vi "Peregrine_close.vi"(2 "error in (no error)":errorcluster, 3 "Handle in":refnum<visa-resource-name>) -> (0 "error out":errorcluster)   [LabVIEW 2019]
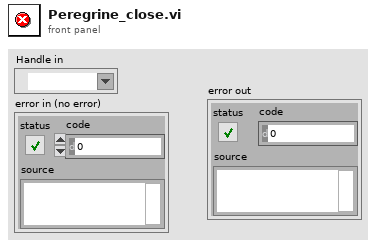
[diagram p1: front panel]
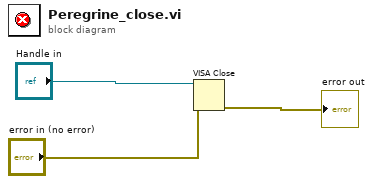
[diagram p0: block diagram]
diagram:
  n1 = VISA Close(VISA resource name="Handle in", error in (no error)="error in (no error)") -> (error out=→"error out":errorcluster)
